vi "CONTROL DBC Functions FGV.vi"(7 "Enum":T1=enum."Set Data", 8 "error in (no error)":errorcluster, 9 "PADDLE IN":string, 10 "TORQUE IN":string, 11 "SPEED IN":string) -> (0 "error out":errorcluster, 1 "PADDLE OUT":string, 2 "TORQUE OUT":string, 3 "SPEED OUT":string)   [LabVIEW 2018]
uses:
  Read File Data.ctl
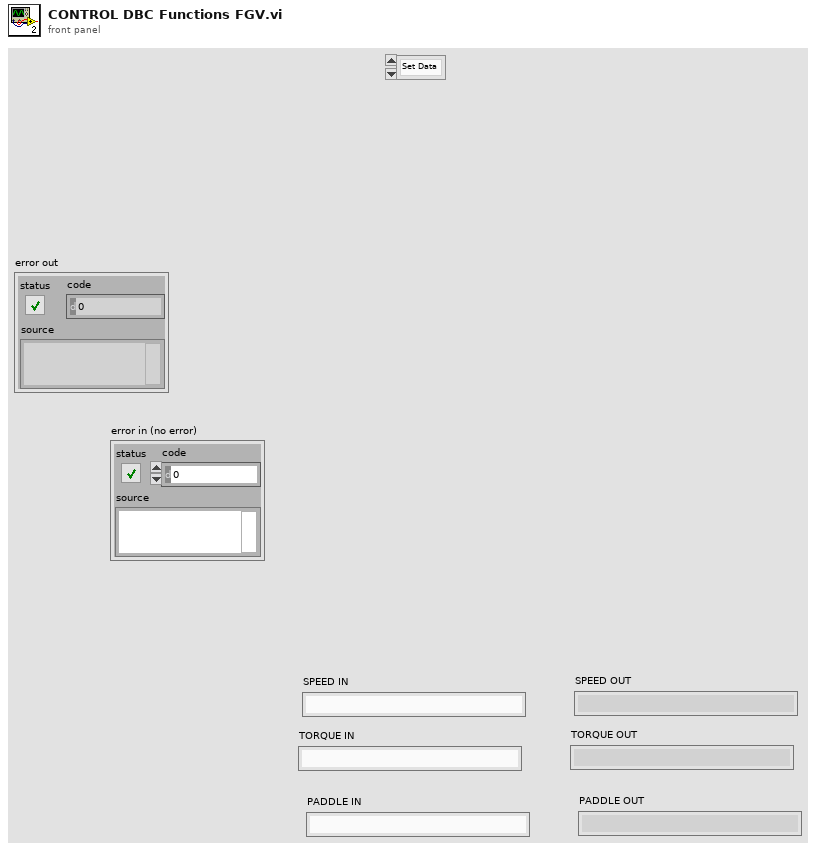
[diagram p1: front panel]
types:
  T1 = typedef "Read File Data.ctl" = enum16{"Get Data", "Set Data"}
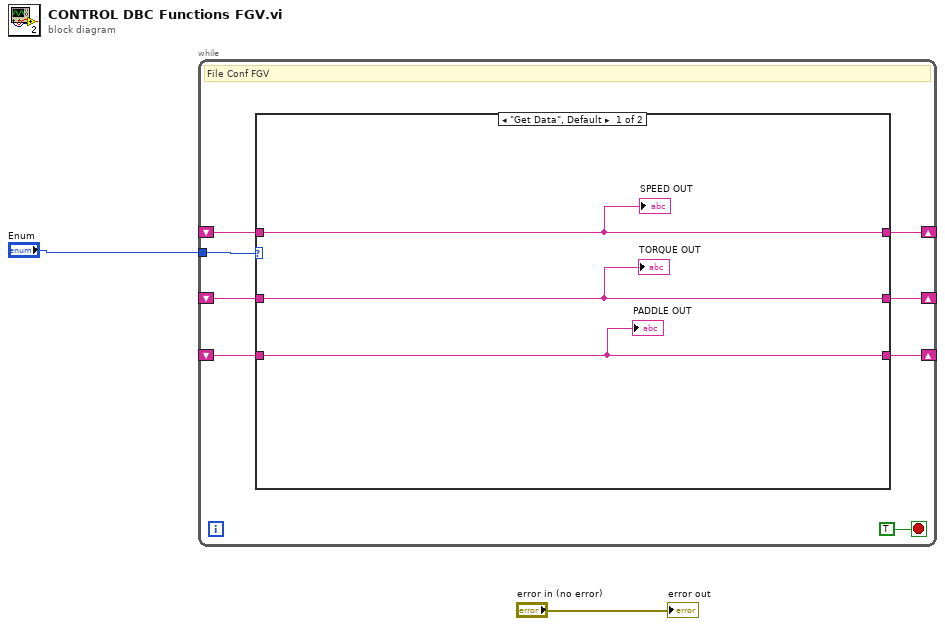
[diagram p0: block diagram]
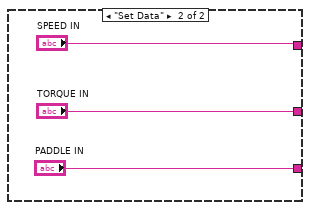
[diagram p2: hidden frame]
diagram:
  n1 = while {
    shift-right: [w9] -> _
    shift-left: _ -> [w8]
    tunnel: "Enum" -> [w7]
    shift-right: [w6] -> _
    shift-left: _ -> [w5]
    shift-right: [w4] -> _
    shift-left: _ -> [w3]
    stop <- TRUE stop-if-true
    # "File Conf FGV"
    n2 = case shown="\"Get Data\", Default" w7 {
      tunnel: [w13 "SPEED IN"] -> w9
      tunnel: w8 -> [w13 _]
      tunnel: [w12 "TORQUE IN"] -> w6
      tunnel: w5 -> [w12 _]
      tunnel: [w11 "PADDLE IN"] -> w4
      tunnel: w3 -> [w11 _]
      frame "Get Data", Default {
        "SPEED OUT" <- w13
        "TORQUE OUT" <- w12
        "PADDLE OUT" <- w11
      }
      frame "Set Data" {
      }
    }
  }
  "error out" <- "error in (no error)"
